vi "Set Status.vi"(8 "error in (no error)":errorcluster, 10 "Success?":bool, 11 "Project Builder in":refnum<class "Project Builder.lvclass">) -> (0 "error out":errorcluster, 3 "Project Builder out":refnum<class "Project Builder.lvclass">)   [LabVIEW 2020, in "ProjectBuilder.lvlib" / "Project Builder.lvclass"]
uses:
  Project Builder.lvclass
  <vilib>/Utility/file.llb/Write Delimited Spreadsheet (string).vi
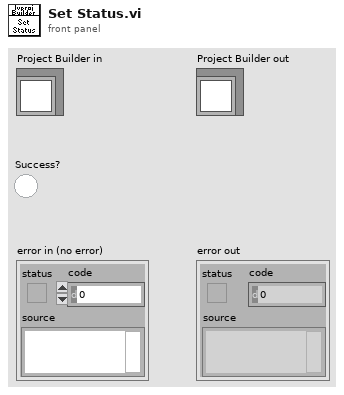
[diagram p1: front panel]
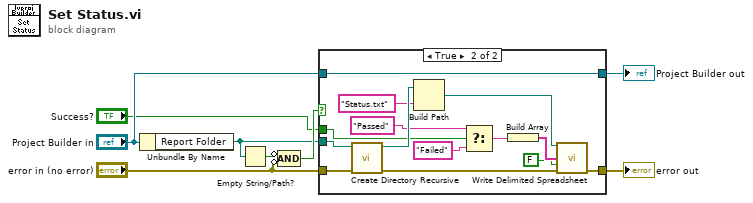
[diagram p0: block diagram]
diagram:
  n1 = Unbundle By Name("Project Builder in") -> ("Report Folder"=w1:path)
  n2 = Empty String/Path?(string/path=w1) -> (empty?=w5:bool)
  n3 = Compound Arithmetic op=AND(invert w5, invert "error in (no error)") -> (w3:bool)
  n4 = case shown="True" w3 {
    tunnel: [w10 w12] -> w8
    tunnel: [w9 w24] -> w6
    tunnel: "Project Builder in" -> [w9 w24]
    tunnel: "error in (no error)" -> [w10 w22]
    tunnel: "Success?" -> [_ w18]
    tunnel: w1 -> [_ w23]
    frame False {
    }
    frame True {
      n5 = call <vilib>:"Create Directory Recursive.vi"("error in (no error)"=w22, "directory"=w23) -> ("error out"=w13:errorcluster, "directory copy"=w21:path)  [unwired: 3 in, 1 out]
      n6 = Build Path(base path=w21, name or relative path="Status.txt") -> (appended path=w19:path)
      n7 = Select(t="Passed", s=w18, f="Failed") -> (s? t:f=w15:string)
      n8 = Build Array(w15) -> (w14:string[])
      n9 = call-poly <vilib>:"Write Delimited Spreadsheet.vi"("file path (dialog if empty)"=w19, "1D data"=w14, "append to file? (new file:F)"=FALSE, "error in (no error)"=w13) -> ("error out"=w12:errorcluster)  [unwired: 10 in, 1 out]
    }
  }
  "error out" <- w8
  "Project Builder out" <- w6
